vi "GetErrorMsg.vi"(4 "error in (no error)":errorcluster, 6 "DeviceKey In":string, 7 "CmdLib In":refnum<k24>) -> (0 "error out":errorcluster, 2 "DeviceKey Out":string, 3 "CmdLib Out":refnum<k24>)   [LabVIEW 2013]
uses:
  C:/Users/Saffmanlab/Documents/git/CsPyController/labview/cesium_controller/PicoMotor/NewFocus8742/CmdLib.dll
  CmdLib.dll
panel:
  in  "message":string
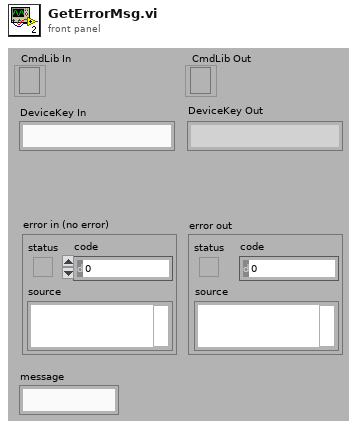
[diagram p1: front panel]
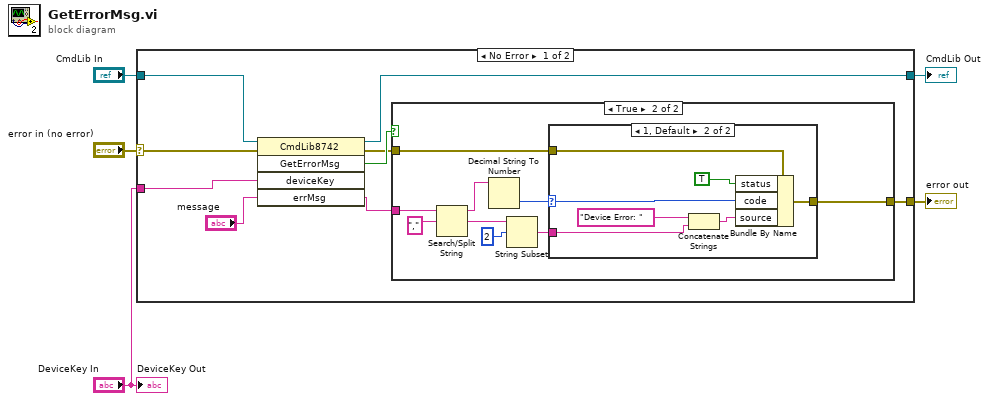
[diagram p0: block diagram]
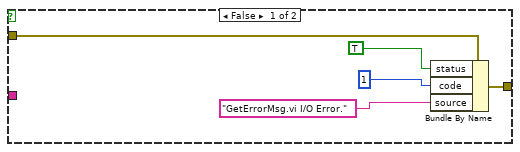
[diagram p2: hidden frame]
diagram:
  n1 = case shown="No Error" "error in (no error)" {
    selector: "error in (no error)" -> [w11 w37]
    tunnel: "CmdLib In" -> [w14 w38]
    tunnel: [w13 w38] -> w4
    tunnel: "DeviceKey In" -> [w12 _]
    tunnel: [w8 w37] -> w1
    frame No Error {
      n2 = invoke class="CmdLib8742" method="GetErrorMsg"(reference=w14, error in=w11, "deviceKey"=w12, "errMsg"="message") -> (reference out=w13:refnum<k24>, error out=w9:errorcluster, "GetErrorMsg"=w10:bool, "errMsg"=w6:string)  [unwired: 1 in, 1 out]
      n3 = case shown="True" w10 {
        tunnel: w9 -> [w19 w22]
        tunnel: [w18 w20] -> w8
        tunnel: w6 -> [_ w28]
        frame False {
          n4 = Bundle By Name(cluster=w19, "status"=TRUE, "code"=1, "source"="GetErrorMsg.vi I/O Error.") -> (w18:errorcluster)
        }
        frame True {
          n5 = Search/Split String(string=w28, search string/char (-)=",") -> (substring before match=w26:string, match + rest of string=w25:string)  [unwired: 1 in, 1 out]
          n6 = Decimal String To Number(string=w26) -> (number=w23:i32)  [unwired: 2 in, 1 out]
          n7 = String Subset(string=w25, offset (0)=2) -> (substring=w21:string)  [unwired: 1 in]
          n8 = case shown="1, Default" w23 {
            selector: w23 -> [_ w34]
            tunnel: w22 -> [w29 w35]
            tunnel: w21 -> [_ w32]
            tunnel: [w29 w33] -> w20
            frame 0 {
            }
            frame 1, Default {
              n9 = Concatenate Strings("Device Error: " ("string"), w32) -> (w31:string)
              n10 = Bundle By Name(cluster=w35, "status"=TRUE, "code"=w34, "source"=w31) -> (w33:errorcluster)
            }
          }
        }
      }
    }
    frame Error {
    }
  }
  "error out" <- w1
  "CmdLib Out" <- w4
  "DeviceKey Out" <- "DeviceKey In"
